vi "Request UI Display--helper.vi"(7 "This Application":refnum<vi>, 8 "error in (no error)":errorcluster, 9 "Display Scenario":T1, 11 "Module DQMH Path":path) -> (0 "error out":errorcluster)   [LabVIEW 2020, in "Navigation.lvlib"]
doc: "____\nHAMPEL SOFTWARE ENGINEERING v2.6.0 (2023-12-19 10:54)"
uses:
  Navigation.lvlib
  Libraries/hse-libraries/Source/hse-dqmh/Controls/Module Display Scenarios.ctl
  Libraries/hse-libraries/Source/hse-dqmh/hse-dqmh.lvlib
  Libraries/hse-libraries/Source/hse-dqmh/hse-dqmh-dynamicrequesters.lvlib
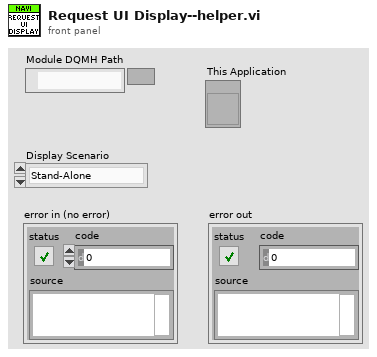
[diagram p1: front panel]
types:
  T1 = typedef "hse-dqmh.lvlib/Module Display Scenarios.ctl" = enum16{"Stand-Alone", "Managed"}
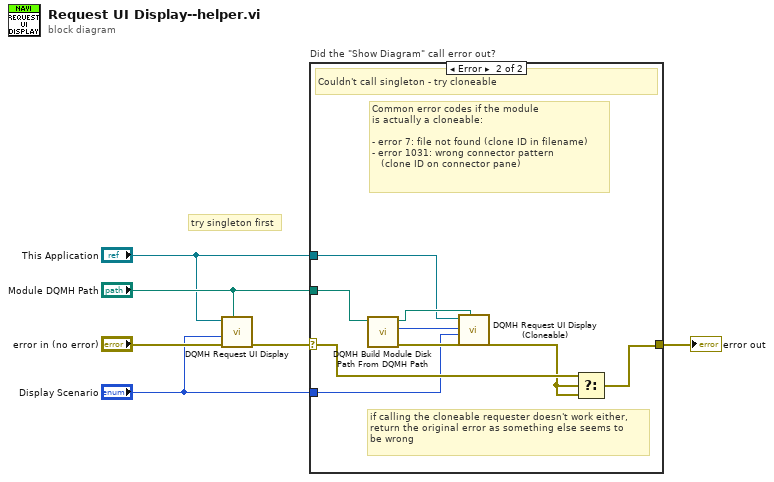
[diagram p0: block diagram]
diagram:
  # "try singleton first"
  n1 = call "DQMH Request UI Display.vi"("Module DIsk Path"="Module DQMH Path", "error in (no error)"="error in (no error)", "Display Scenario"="Display Scenario", "Application reference"="This Application") -> ("error out"=w3:errorcluster)  [unwired: 6 in, 1 out]
  n2 = case "Did the \"Show Diagram\" call error out?" shown="Error" w3 {
    selector: w3 -> [w7 w15]
    tunnel: "Module DQMH Path" -> [_ w16]
    tunnel: "This Application" -> [_ w9]
    tunnel: [w7 w14] -> w6
    tunnel: "Display Scenario" -> [_ w8]
    frame No Error {
    }
    frame Error {
      # "if calling the cloneable requester doesn't work either,\nreturn the original error as something else seems to \nbe wrong"
      # "Common error codes if the module \nis actually a cloneable:\n\n- error 7: file not found (clone ID in filename)\n- error 1031: wrong connector pattern \n   (clone ID on connector pane)"
      # "Couldn't call singleton - try cloneable"
      n3 = call "DQMH Build Module Disk Path From DQMH Path.vi"("Module DQMH Path"=w16) -> ("error out"=w11:errorcluster, "Clone ID"=w12:i32, "Module Disk Path"=w10:path)  [unwired: 7 in, 1 out]
      n4 = call "DQMH Request UI Display (Cloneable).vi"("Module Disk Path"=w10, "error in (no error)"=w11, "Display Scenario"=w8, "Module ID"=w12, "Application reference"=w9) -> ("error out"=w13:errorcluster)  [unwired: 5 in, 1 out]
      n5 = Select(t=w15, s=w13, f=w13) -> (s? t:f=w14:errorcluster)
    }
  }
  "error out" <- w6
